vi "ExposeMapperDataValueToWaveform.vi"(11 "Data Value Reference in":refnum<data-value>) -> (3 "Data Value Reference out":refnum<data-value>)   [LabVIEW 2017]
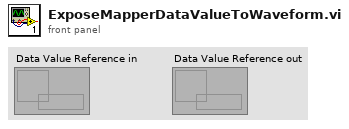
[diagram p1: front panel]
types:
  T1 = typedef "ExposeObjectMapContainerTypeEnum.ctl" = enum16{"Value", "Array", "Waveform", "NetContainer"}
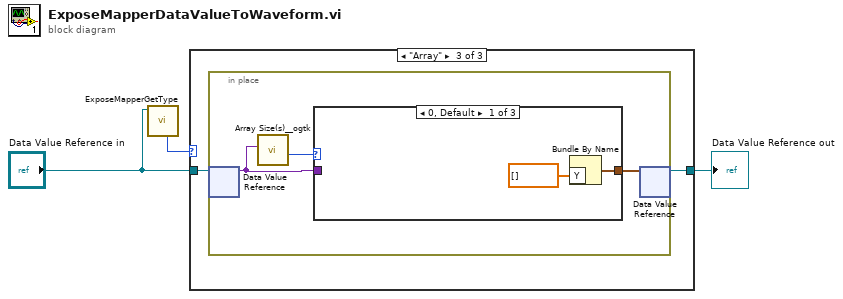
[diagram p0: block diagram]
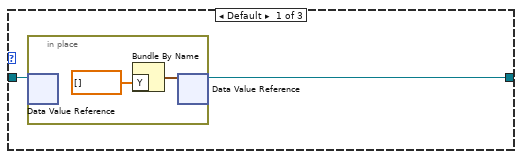
[diagram p2: hidden frame]
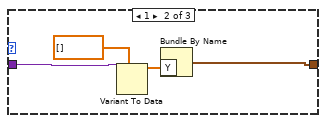
[diagram p4: hidden frame]
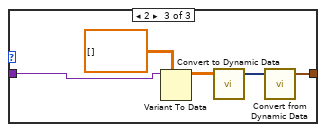
[diagram p5: hidden frame]
diagram:
  n1 = call "ExposeMapperGetType.vi"("Data Val Ref in"="Data Value Reference in") -> ("Container Type (Labview Value type)"=w1:T1)  [unwired: 5 in, 5 out]
  n2 = case shown="\"Array\"" w1 {
    tunnel: [w5 w8 w9] -> w3
    tunnel: "Data Value Reference in" -> [w4 w8 w10]
    frame Default {
      n3 = in-place {
        n4 = in-place-dvr #1(w4) -> ()  [unwired: 2 out]
        n5 = Bundle By Name("Y"=dbl[] []) -> (w6:waveform(dbl))  [unwired: 1 in]
        n6 = in-place-dvr #1(w6) -> (w5:refnum<data-value>)  [unwired: 1 out]
      }
    }
    frame "Waveform" {
    }
    frame "Array" {
      n7 = in-place {
        n8 = in-place-dvr #2(w10) -> (w11:variant)  [unwired: 1 out]
        n9 = call <userlib>:"Array Size(s)__ogtk.vi"("Array"=w11) -> ("N dims"=w13:u32)  [unwired: 8 in, 2 out]
        n10 = case shown="0, Default" w13 {
          tunnel: [w14 w16 w20] -> w12
          tunnel: w11 -> [_ w18 w24]
          frame 0, Default {
            n11 = Bundle By Name("Y"=dbl[] []) -> (w14:waveform(dbl))  [unwired: 1 in]
          }
          frame 1 {
            n12 = Variant To Data(type=dbl[] [] ("Y"), Variant=w18) -> (data=w17:dbl[])  [unwired: 1 in, 1 out]
            n13 = Bundle By Name("Y"=w17) -> (w16:waveform(dbl))  [unwired: 1 in]
          }
          frame 2 {
            n14 = Variant To Data(type=dbl[][] [] ("Y"), Variant=w24) -> (data=w22:dbl[][])  [unwired: 1 in, 1 out]
            n15 = call "Convert to Dynamic Data"("2D Array"=w22) -> ("Dynamic Data Type"=w21:dynamicdata)  [unwired: 3 in]
            n16 = call "Convert from Dynamic Data"("Dynamic Data Type"=w21) -> ("Waveform"=w20:waveform(dbl))  [unwired: 3 in]
          }
        }
        n17 = in-place-dvr #2(w12) -> (w9:refnum<data-value>)  [unwired: 1 out]
      }
    }
  }
  "Data Value Reference out" <- w3
